vi "Write x offset for waveform.vi"   [LabVIEW 2025]
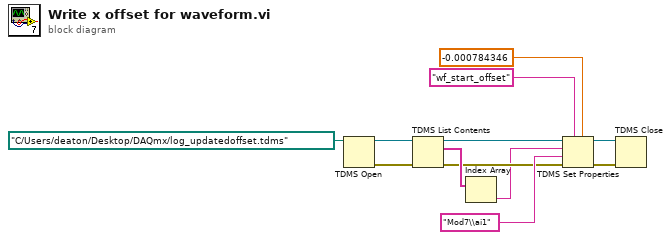
[diagram p0: block diagram]
diagram:
  n1 = TDMS Open(11:path "C:/Users/deaton/Desktop/DAQmx/log_updatedoffset.tdms" ("file path")) -> (0:w6:errorcluster, 3:w7:refnum<k34>)  [unwired: 6 in]
  n2 = TDMS List Contents(4:w6, 7:w7) -> (0:w3:errorcluster, 2:w5:string[], 3:w2:refnum<k34>)  [unwired: 1 in, 1 out]
  n3 = Index Array(array=w5) -> (element=w1:string)  [unwired: 1 in]
  n4 = TDMS Set Properties(5:-0.000784346, 7:"wf_start_offset" ("group name in"), 8:w3, 9:"Mod7\\ai1", 10:w1, 11:w2) -> (0:w9:errorcluster, 3:w10:refnum<k34>)  [unwired: 2 out]
  n5 = TDMS Close(8:w9, 11:w10) -> ()  [unwired: 2 out]
